vi "GetMACAddress.vi"() -> (0 "MAC Address":string)   [LabVIEW 2020]
doc: "This VI uses the system exec VI to issue the command line utilities \"ping\" and \"arp\" to obtain the MAC Address of the network interface from a different computer on your network. Its functionality is limited to Windows systems.\n\nThe arp utility only works for IP addresses on the same local subnet as the computer executing the VI. Furthermore, it does not work for the IP address of the computer running the VI. This utility attempts to use the ipconfig utility for Windows NT/2000/XP to get the MAC Address of the local computer, but if the local computer's IP Address is given, it will fail when run under Windows 9x or Windows ME."
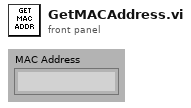
[diagram p1: front panel]
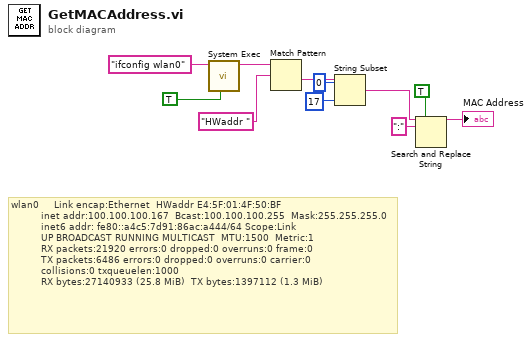
[diagram p0: block diagram]
diagram:
  # "wlan0     Link encap:Ethernet  HWaddr E4:5F:01:4F:50:BF  \n          inet addr:100.100.100.167  Bcast:100.100.100.255  Mask:255.255.255.0\n          inet6 addr: fe80::a4c5:7d91:86ac:a444/64 Scope:Link\n          UP BROADCAST RUNNING MULTICAST  MTU:1500  Metric:1\n          RX packets:21920 errors:0 dropped:0 overruns:0 frame:0\n          TX packets:6486 errors:0 dropped:0 overruns:0 carrier:0\n          collisions:0 txqueuelen:1000 \n          RX bytes:27140933 (25.8 MiB)  TX bytes:1397112 (1.3 MiB)"
  n1 = call <vilib>:"System Exec.vi"("run minimized? (F)"=TRUE, "command line"="ifconfig wlan0") -> ("standard output"=w9:string)  [unwired: 4 in, 5 out]
  n2 = Match Pattern(string=w9, regular expression="HWaddr ") -> (after substring=w8:string)  [unwired: 4 out]
  n3 = String Subset(string=w8, offset (0)=0, length (rest)=17 ("length (rest)")) -> (substring=w4:string)
  n4 = Search and Replace String(replace all?=TRUE ("replace all? (F)"), input string=w4, search string=":") -> (result string=→"MAC Address":string)  [unwired: 5 in, 3 out]
